vi "MB ICPCON Registers Write DW.vi"(7 "Data Reference":T1, 8 "error in (no error)":errorcluster, 9 "Bits In":bool[](array[boolean]), 11 "N":i32) -> (0 "error out":errorcluster)   [LabVIEW 2019, in "ICPCON Registers.lvlib"]
uses:
  ICPCON Registers.lvlib
  Ctl/ICPCON Data.ctl
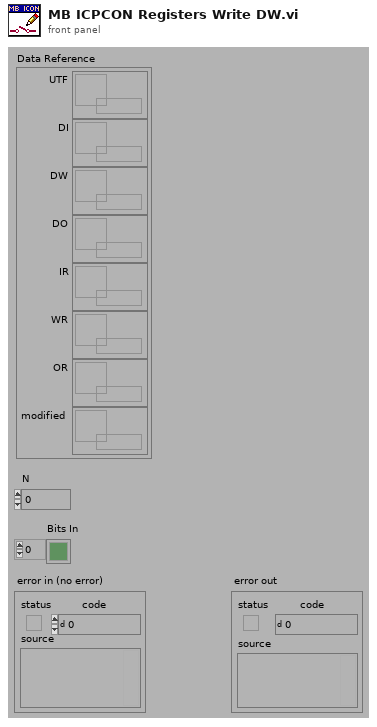
[diagram p1: front panel]
types:
  T1 = typedef "ICPCON Registers.lvlib/ICPCON Data.ctl" = cluster{"UTF":refnum<data-value>, "DI":refnum<data-value>, "DW":refnum<data-value>, "DO":refnum<data-value>, "IR":refnum<data-value>, "WR":refnum<data-value>, "OR":refnum<data-value>, "modified":refnum<data-value>}
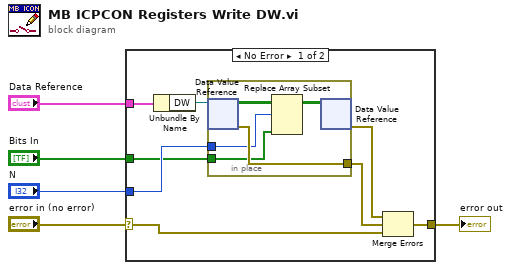
[diagram p0: block diagram]
diagram:
  n1 = case shown="No Error" "error in (no error)" {
    selector: "error in (no error)" -> [w6 w19]
    tunnel: [w11 w19] -> w3
    tunnel: "N" -> [w13 _]
    tunnel: "Data Reference" -> [w12 _]
    tunnel: "Bits In" -> [w10 _]
    frame No Error {
      n2 = Unbundle By Name(w12) -> ("DW"=w7:refnum<data-value>)
      n3 = in-place {
        in-place-border: w13 -> [w15]
        in-place-border: [w18] -> w8
        in-place-border: w10 -> [w14]
        n4 = in-place-dvr #1(w7) -> (w17:bool[][], w18:errorcluster)
        n5 = Replace Array Subset(array=w17, new element=w14, index (row)=w15) -> (w16:bool[][])  [unwired: 1 in]
        n6 = in-place-dvr #1(w16) -> (w9:errorcluster)  [unwired: 1 out]
      }
      n7 = Merge Errors(w9, w8, w6) -> (w11:errorcluster)
    }
    frame Error {
    }
  }
  "error out" <- w3
